vi "Laser_control.vi"() -> ()   [LabVIEW 2011]
panel:
  in  "Power":dbl(knob)=100.0 min=0.0 max=100.0 step=5.0 scale=0.0..100.0 scale format="%#_3g"
  in  "is on?":bool
  out "Power set":dbl(knob) scale=0.0..100.0 scale format="%#_3g"
  out "Photodiode":i32(knob) scale=0.0..20.0 scale format="%-3.0f"
  out "Backreflection":i32(knob) scale=0.0..500.0
  out "Amplifier":i32[](graph)
  out "Preamplifier":i32(knob) scale=0.0..4500.0
  out "Laser Temperature":dbl[](graph)
  out "Time to go":i32
  in  "Power down":bool
  in  "Power Button":bool
  out "Laser Connected":bool
  out "Laser ready":bool
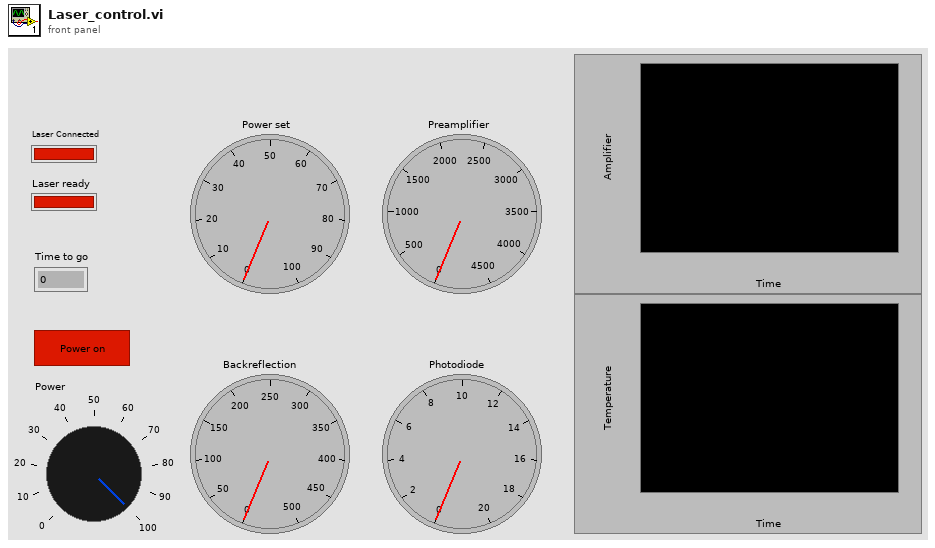
[diagram p1: front panel]
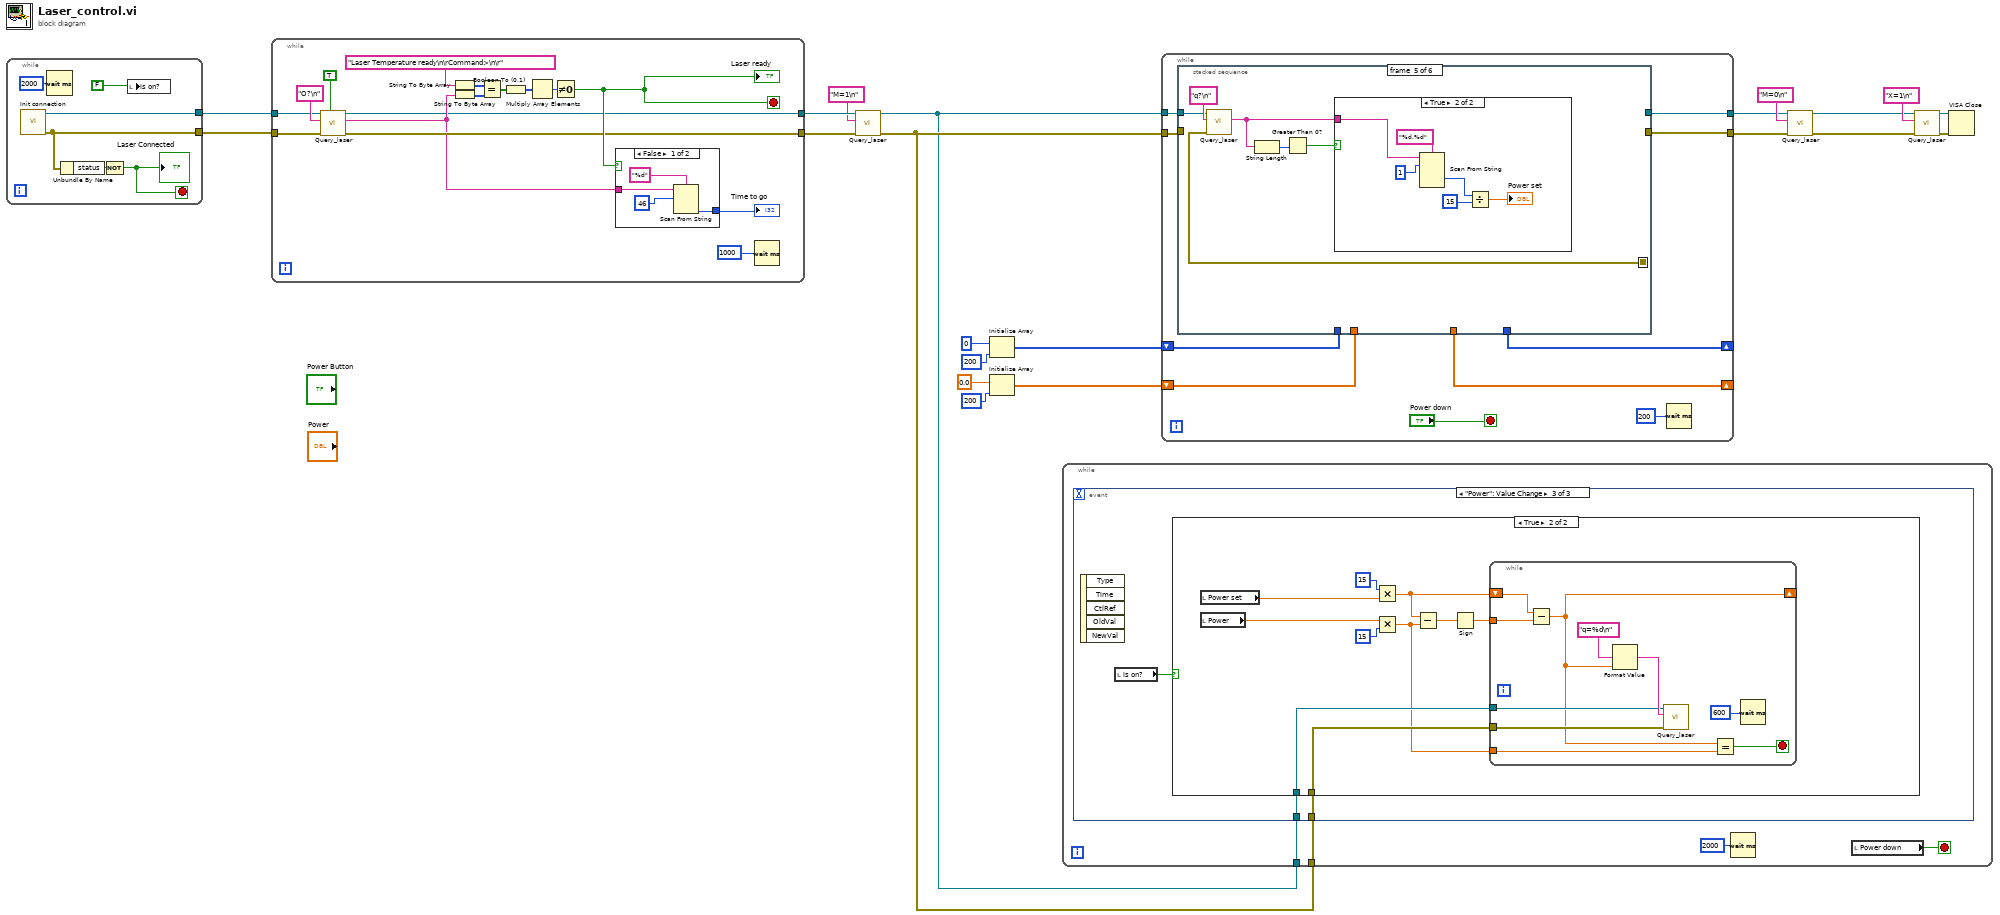
[diagram p0: block diagram]
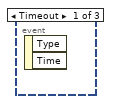
[diagram p2: hidden frame]
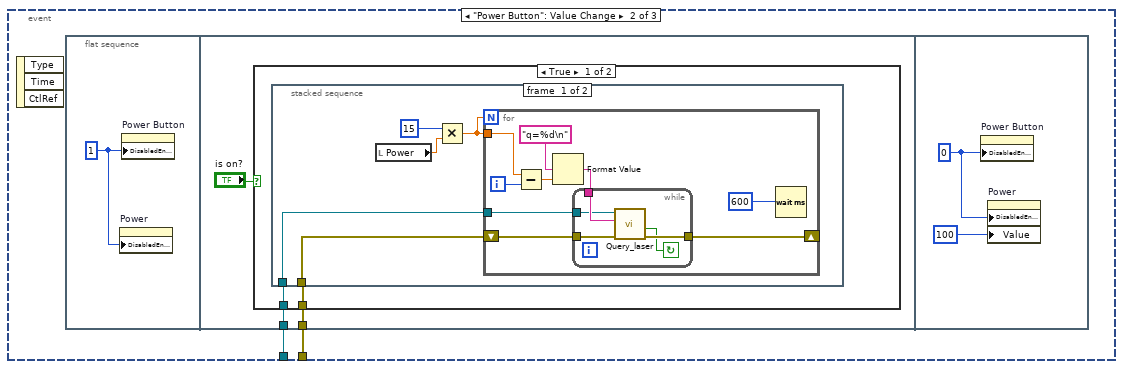
[diagram p3: hidden frame]
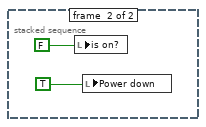
[diagram p4: hidden frame]
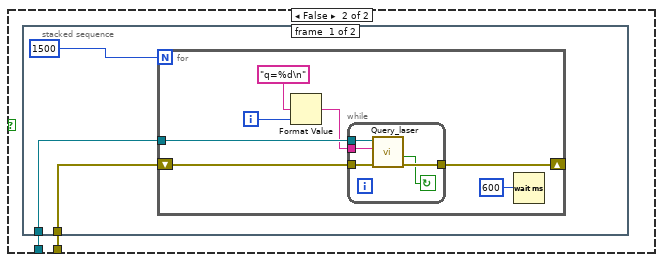
[diagram p5: hidden frame]
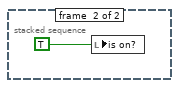
[diagram p6: hidden frame]
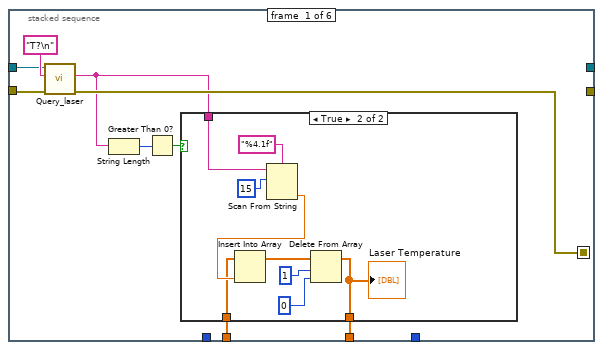
[diagram p8: hidden frame]
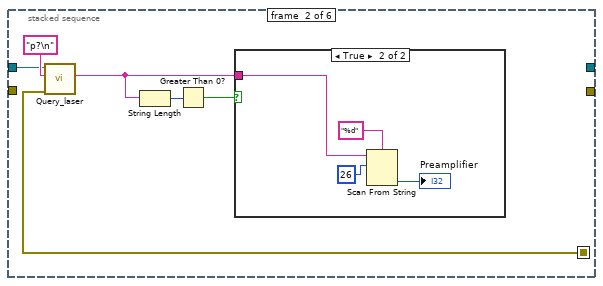
[diagram p10: hidden frame]
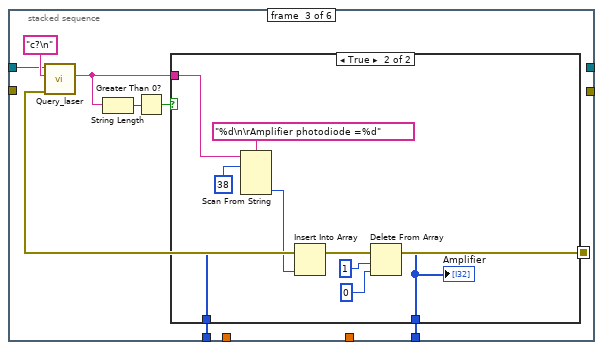
[diagram p12: hidden frame]
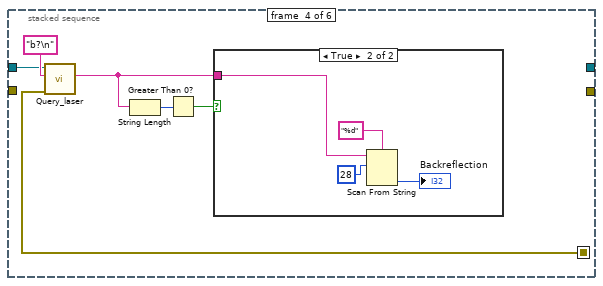
[diagram p14: hidden frame]
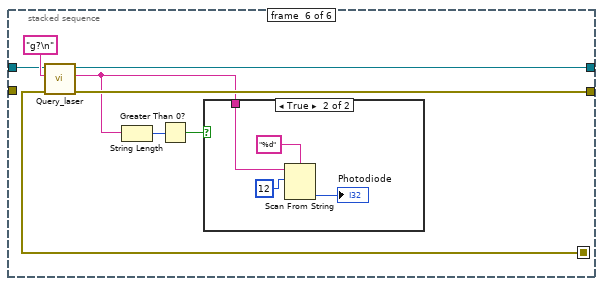
[diagram p17: hidden frame]
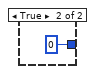
[diagram p19: hidden frame]
diagram:
  n1 = while {
    tunnel: [w25] -> w1
    tunnel: [w24] -> w2
    stop <- w23 stop-if-true
    n2 = call "Init connection.vi"() -> ("error constant"=w25:errorcluster, "VISA resource name 2"=w24:refnum<visa-resource-name>)  [unwired: 10 in]
    n3 = Wait (ms)(milliseconds to wait=2000) -> ()  [unwired: 1 out]
    n4 = Unbundle By Name(w25) -> ("status"=w26:bool)
    n5 = Not(x=w26) -> (.not. x?=w23:bool)
    "Laser Connected" <- w23
    n6 = local write "is on?"(FALSE) -> ()
  }
  n7 = while {
    tunnel: w2 -> [w41]
    tunnel: w1 -> [w40]
    tunnel: [w29] -> w5
    tunnel: [w31] -> w7
    stop <- w33 stop-if-true
    n8 = call "Query_laser.vi"("Reset?"=TRUE, "error in (no error)"=w40, "String in"="O?\n", "VISA resource name"=w41) -> ("error out"=w31:errorcluster, "String out"=w30:string, "VISA resource name 2"=w29:refnum<visa-resource-name>)  [unwired: 3 in, 1 out]
    n9 = String To Byte Array(string="Laser Temperature ready\n\rCommand>\n\r") -> (unsigned byte array=w38:u8[])
    n10 = String To Byte Array(string=w30) -> (unsigned byte array=w37:u8[])
    n11 = Equal?(x=w38, y=w37) -> (x = y?=w36:bool[])
    n12 = Boolean To (0,1)(Boolean=w36) -> (0, 1=w35:i16[])
    n13 = Multiply Array Elements(1:w35) -> (0:w34:i16)
    n14 = Not Equal To 0?(x=w34) -> (x != 0?=w33:bool)
    "Laser ready" <- w33
    n15 = case shown="False" w33 {
      tunnel: w30 -> [w47 _]
      tunnel: [w45 0] -> w32
      frame False {
        n16 = Scan From String(format string="%d", input string=w47, initial scan location=46) -> (output 1=w45:i32)  [unwired: 2 in, 3 out]
      }
      frame True {
      }
    }
    "Time to go" <- w32
    n17 = Wait (ms)(milliseconds to wait=1000) -> ()  [unwired: 1 out]
  }
  n18 = call "Query_laser.vi"("error in (no error)"=w7, "String in"="M=1\n", "VISA resource name"=w5) -> ("error out"=w6:errorcluster, "VISA resource name 2"=w4:refnum<visa-resource-name>)  [unwired: 4 in, 2 out]
  n19 = Initialize Array(0, 200) -> (w8:i32[])
  n20 = Initialize Array(0.0, 200) -> (w11:dbl[])
  n21 = while {
    tunnel: w6 -> [w52]
    tunnel: w4 -> [w51]
    stop <- w50 stop-if-true
    n22 = event shown="[2] \"Power\": Value Change" {
      selector: _ -> [_ _ _]
      dyn-events: _ -> [_ _ _]
      timeout: _ -> [_ _ _]
      tunnel: w52 -> [_ w54 w103]
      tunnel: w51 -> [_ w53 w102]
      event Timeout {
        n23 = event-data() -> ()  [unwired: 1 in, 2 out]
      }
      event "Power Button": Value Change {
        n24 = event-data() -> ()  [unwired: 1 in, 3 out]
        n25 = flat-sequence {
          tunnel: w53 -> [w58]
          tunnel: w54 -> [w57]
          frame #0 {
            w55 = 1
            n26 = property on="Power" class="Knob (strict)"("DisabledEnum"=w55) -> ()  [unwired: 2 in, 2 out]
            n27 = property on="Power Button" class="Bool (strict)"("DisabledEnum"=w55) -> ()  [unwired: 2 in, 2 out]
          }
          frame #1 {
            n28 = case shown="True" "is on?" {
              tunnel: w57 -> [w60 w83]
              tunnel: w58 -> [w59 w82]
              frame True {
                n29 = stacked-sequence {
                  tunnel: w60 -> [w65 _]
                  tunnel: w59 -> [w64 _]
                  frame #0 {
                    n30 = local read "Power"() -> (w62:dbl)
                    n31 = Multiply(x=15, y=w62) -> (x*y=w61:dbl)
                    n32 = for {
                      N: w61 -> [_]
                      shift-right: [w69] -> _
                      shift-left: w65 -> [w71]
                      tunnel: w64 -> [w70]
                      tunnel: w61 -> [w66]
                      i -> [w68]
                      n33 = Subtract(x=w66, y=w68) -> (x-y=w67:dbl)
                      n34 = Format Value(format string="q=%d\n", value (0)=w67) -> (output string=w72:string)  [unwired: 1 in]
                      n35 = while {
                        tunnel: w72 -> [w79]
                        tunnel: w71 -> [w78]
                        tunnel: w70 -> [w77]
                        tunnel: [w76] -> w69
                        stop <- w75 continue-if-true
                        n36 = call "Query_laser.vi"("error in (no error)"=w78, "String in"=w79, "VISA resource name"=w77) -> ("error out"=w76:errorcluster, "was busy?"=w75:bool)  [unwired: 4 in, 2 out]
                      }
                      n37 = Wait (ms)(milliseconds to wait=u32 600) -> ()  [unwired: 1 out]
                    }
                  }
                  frame #1 {
                    n38 = local write "is on?"(FALSE) -> ()
                    n39 = local write "Power down"(TRUE) -> ()
                  }
                }
              }
              frame False {
                n40 = stacked-sequence {
                  tunnel: w83 -> [w85 _]
                  tunnel: w82 -> [w84 _]
                  frame #0 {
                    n41 = for {
                      N: 1500 -> [_]
                      shift-right: [w88] -> _
                      shift-left: w85 -> [w90]
                      tunnel: w84 -> [w91]
                      i -> [w87]
                      n42 = Format Value(format string="q=%d\n", value (0)=w87) -> (output string=w89:string)  [unwired: 1 in]
                      n43 = while {
                        tunnel: w91 -> [w98]
                        tunnel: w90 -> [w97]
                        tunnel: w89 -> [w96]
                        tunnel: [w95] -> w88
                        stop <- w94 continue-if-true
                        n44 = call "Query_laser.vi"("error in (no error)"=w97, "String in"=w96, "VISA resource name"=w98) -> ("error out"=w95:errorcluster, "was busy?"=w94:bool)  [unwired: 4 in, 2 out]
                      }
                      n45 = Wait (ms)(milliseconds to wait=u32 600) -> ()  [unwired: 1 out]
                    }
                  }
                  frame #1 {
                    n46 = local write "is on?"(TRUE) -> ()
                  }
                }
              }
            }
          }
          frame #2 {
            w101 = 0
            n47 = property on="Power Button" class="Bool (strict)"("DisabledEnum"=w101) -> ()  [unwired: 2 in, 2 out]
            n48 = property on="Power" class="Knob (strict)"("DisabledEnum"=w101, "Value"=100) -> ()  [unwired: 2 in, 2 out]
          }
        }
      }
      event "Power": Value Change {
        n49 = event-data() -> ()  [unwired: 1 in, 5 out]
        n50 = local read "is on?"() -> (w104:bool)
        n51 = case shown="True" w104 {
          tunnel: w103 -> [_ w110]
          tunnel: w102 -> [_ w111]
          frame False {
          }
          frame True {
            n52 = local read "Power set"() -> (w113:dbl)
            n53 = local read "Power"() -> (w105:dbl)
            n54 = Multiply(x=15, y=w113) -> (x*y=w107:dbl)
            n55 = Multiply(x=w105, y=15) -> (x*y=w108:dbl)
            n56 = Subtract(x=w107, y=w108) -> (x-y=w109:dbl)
            n57 = Sign(1:w109) -> (0:w106:dbl)
            n58 = while {
              tunnel: w111 -> [w121]
              tunnel: w110 -> [w120]
              tunnel: w108 -> [w118]
              shift-right: [w115] -> _
              shift-left: w107 -> [w117]
              tunnel: w106 -> [w116]
              stop <- w119 stop-if-true
              n59 = Subtract(x=w117, y=w116) -> (x-y=w115:dbl)
              n60 = Format Value(format string="q=%d\n", value (0)=w115) -> (output string=w123:string)  [unwired: 1 in]
              n61 = call "Query_laser.vi"("error in (no error)"=w120, "String in"=w123, "VISA resource name"=w121) -> ()  [unwired: 4 in, 4 out]
              n62 = Equal?(x=w115, y=w118) -> (x = y?=w119:bool)
              n63 = Wait (ms)(milliseconds to wait=u32 600) -> ()  [unwired: 1 out]
            }
          }
        }
      }
    }
    n64 = Wait (ms)(milliseconds to wait=u32 2000) -> ()  [unwired: 1 out]
    n65 = local read "Power down"() -> (w50:bool)
  }
  n66 = while {
    tunnel: w4 -> [w132]
    tunnel: w6 -> [w133]
    tunnel: [w130] -> w15
    tunnel: [w131] -> w14
    shift-right: [w126] -> _
    shift-left: w11 -> [w128]
    shift-right: [w125] -> _
    shift-left: w8 -> [w127]
    stop <- "Power down" stop-if-true
    n67 = stacked-sequence {
      seq-local: [w138 _ _ _ _ _] -> [_ w154 w170 w186 w196 w210]
      tunnel: w132 -> [w141 w158 w167 w185 w195 w207]
      tunnel: w133 -> [w142 _ _ _ _ _]
      tunnel: [_ _ _ _ _ w209] -> w131
      tunnel: [_ _ _ _ _ w208] -> w130
      tunnel: w128 -> [w140 _ _ _ _ _]
      tunnel: w127 -> [_ _ w169 _ _ _]
      tunnel: [w139 _ _ _ _ _] -> w126
      tunnel: [_ _ w168 _ _ _] -> w125
      frame #0 {
        n68 = call "Query_laser.vi"("error in (no error)"=w142, "String in"="T?\n", "VISA resource name"=w141) -> ("error out"=w138:errorcluster, "String out"=w136:string)  [unwired: 4 in, 2 out]
        n69 = String Length(string=w136) -> (length=w137:i32)
        n70 = Greater Than 0?(x=w137) -> (x > 0?=w135:bool)
        n71 = case shown="True" w135 {
          tunnel: w140 -> [w144 w150]
          tunnel: [w144 w146] -> w139
          tunnel: w136 -> [_ w145]
          frame False {
          }
          frame True {
            n72 = Scan From String(format string="%4.1f", input string=w145, initial scan location=15) -> (output 1=w151:dbl)  [unwired: 2 in, 3 out]
            n73 = Insert Into Array(array=w150, new element=w151) -> (w149:dbl[])  [unwired: 1 in]
            n74 = Delete From Array(array=w149, length=1, index=0) -> (array with subset deleted=w146:dbl[])  [unwired: 1 out]
            "Laser Temperature" <- w146
          }
        }
      }
      frame #1 {
        n75 = call "Query_laser.vi"("error in (no error)"=w154, "String in"="p?\n", "VISA resource name"=w158) -> ("String out"=w157:string)  [unwired: 4 in, 3 out]
        n76 = String Length(string=w157) -> (length=w156:i32)
        n77 = Greater Than 0?(x=w156) -> (x > 0?=w155:bool)
        n78 = case shown="True" w155 {
          tunnel: w157 -> [_ w160]
          frame False {
          }
          frame True {
            n79 = Scan From String(format string="%d", input string=w160, initial scan location=26) -> (output 1=→"Preamplifier":i32)  [unwired: 2 in, 3 out]
          }
        }
      }
      frame #2 {
        n80 = call "Query_laser.vi"("error in (no error)"=w170, "String in"="c?\n", "VISA resource name"=w167) -> ("String out"=w164:string)  [unwired: 4 in, 3 out]
        n81 = String Length(string=w164) -> (length=w166:i32)
        n82 = Greater Than 0?(x=w166) -> (x > 0?=w165:bool)
        n83 = case shown="True" w165 {
          tunnel: w169 -> [w172 w175]
          tunnel: [w172 w174] -> w168
          tunnel: w164 -> [_ w173]
          frame False {
          }
          frame True {
            n84 = Scan From String(format string="%d\n\rAmplifier photodiode =%d", input string=w173, initial scan location=38) -> (output 2=w176:i32)  [unwired: 4 in, 3 out]
            n85 = Insert Into Array(array=w175, new element=w176) -> (w179:i32[])  [unwired: 1 in]
            n86 = Delete From Array(array=w179, length=1, index=0) -> (array with subset deleted=w174:i32[])  [unwired: 1 out]
            "Amplifier" <- w174
          }
        }
      }
      frame #3 {
        n87 = call "Query_laser.vi"("error in (no error)"=w186, "String in"="b?\n", "VISA resource name"=w185) -> ("String out"=w183:string)  [unwired: 4 in, 3 out]
        n88 = String Length(string=w183) -> (length=w184:i32)
        n89 = Greater Than 0?(x=w184) -> (x > 0?=w182:bool)
        n90 = case shown="True" w182 {
          tunnel: w183 -> [_ w188]
          frame False {
          }
          frame True {
            n91 = Scan From String(format string="%d", input string=w188, initial scan location=28) -> (output 1=→"Backreflection":i32)  [unwired: 2 in, 3 out]
          }
        }
      }
      frame #4 {
        n92 = call "Query_laser.vi"("error in (no error)"=w196, "String in"="q?\n", "VISA resource name"=w195) -> ("String out"=w193:string)  [unwired: 4 in, 3 out]
        n93 = String Length(string=w193) -> (length=w194:i32)
        n94 = Greater Than 0?(x=w194) -> (x > 0?=w192:bool)
        n95 = case shown="True" w192 {
          tunnel: w193 -> [_ w198]
          frame False {
          }
          frame True {
            n96 = Scan From String(format string="%d,%d", input string=w198, initial scan location=1) -> (output 1=w199:i32)  [unwired: 4 in, 3 out]
            n97 = Divide(x=w199, y=15) -> (x/y=→"Power set":dbl)
          }
        }
      }
      frame #5 {
        n98 = call "Query_laser.vi"("error in (no error)"=w210, "String in"="g?\n", "VISA resource name"=w207) -> ("error out"=w208:errorcluster, "String out"=w205:string, "VISA resource name 2"=w209:refnum<visa-resource-name>)  [unwired: 4 in, 1 out]
        n99 = String Length(string=w205) -> (length=w206:i32)
        n100 = Greater Than 0?(x=w206) -> (x > 0?=w204:bool)
        n101 = case shown="True" w204 {
          tunnel: w205 -> [_ w212]
          frame False {
          }
          frame True {
            n102 = Scan From String(format string="%d", input string=w212, initial scan location=12) -> (output 1=→"Photodiode":i32)  [unwired: 2 in, 3 out]
          }
        }
      }
    }
    n103 = Wait (ms)(milliseconds to wait=u32 200) -> ()  [unwired: 1 out]
  }
  n104 = call "Query_laser.vi"("error in (no error)"=w15, "String in"="M=0\n", "VISA resource name"=w14) -> ("error out"=w16:errorcluster, "VISA resource name 2"=w17:refnum<visa-resource-name>)  [unwired: 4 in, 2 out]
  n105 = call "Query_laser.vi"("error in (no error)"=w16, "String in"="X=1\n", "VISA resource name"=w17) -> ("error out"=w20:errorcluster, "VISA resource name 2"=w19:refnum<visa-resource-name>)  [unwired: 4 in, 2 out]
  n106 = VISA Close(VISA resource name=w19, error in (no error)=w20) -> ()  [unwired: 1 out]
